vi "EXO2 Message.vi"(11 "字符串":string) -> (2 "数组":dbl[](array[numeric]), 3 "EXO message":T1)   [LabVIEW 2016, in "EXO2.lvlib"]
uses:
  EXO2.lvlib
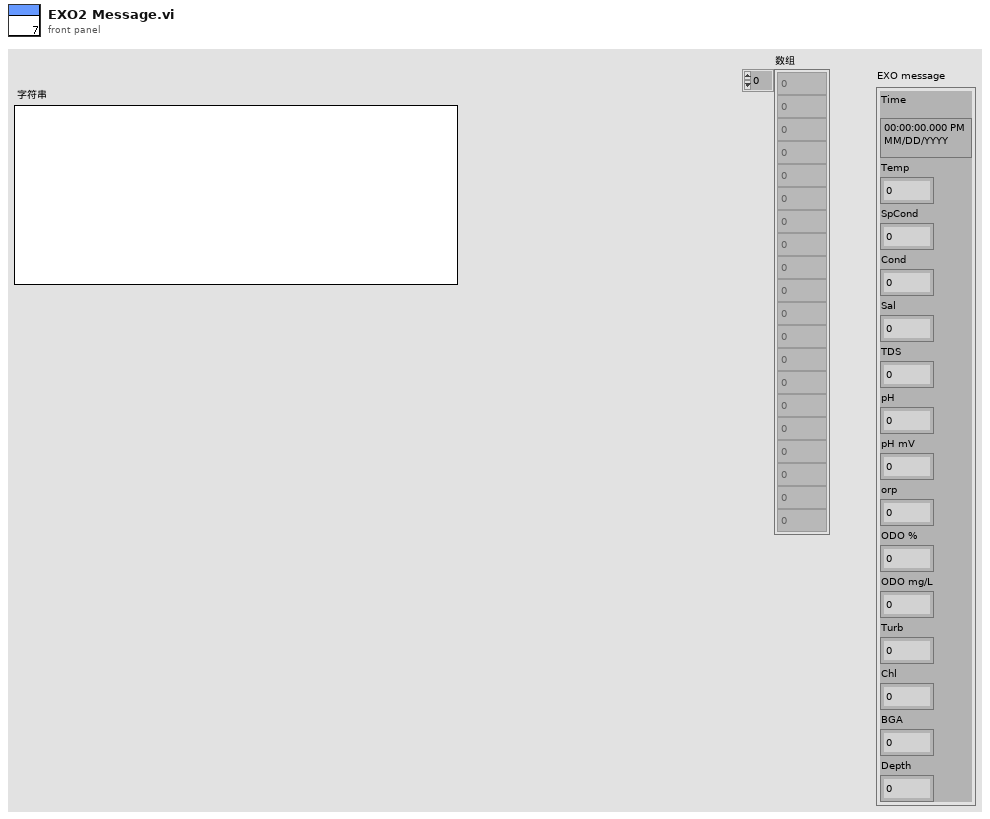
[diagram p1: front panel]
types:
  T1 = cluster{"Time":timestamp, "Temp":dbl, "SpCond":dbl, "Cond":dbl, "Sal":dbl, "TDS":dbl, "pH":dbl, "pH mV":dbl, "orp":dbl, "ODO %":dbl, "ODO mg/L":dbl, "Turb":dbl, "Chl":dbl, "BGA":dbl, "Depth":dbl}
  T2 = cluster{"seconds since 1Jan1904":timestamp, dbl, dbl, dbl, dbl, dbl, dbl, dbl, dbl, dbl, dbl, dbl, dbl, dbl, dbl}
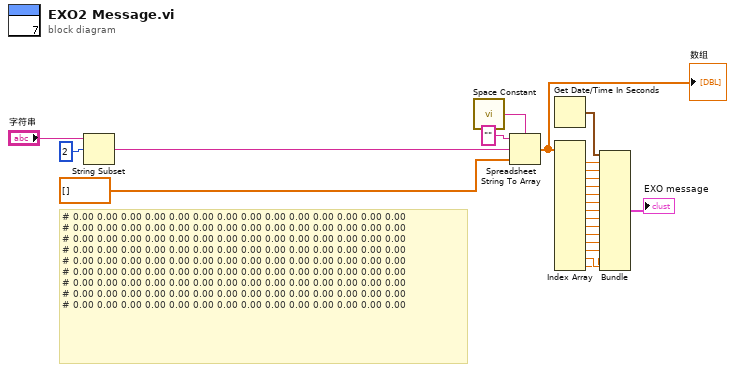
[diagram p0: block diagram]
diagram:
  # "# 0.00 0.00 0.00 0.00 0.00 0.00 0.00 0.00 0.00 0.00 0.00 0.00 0.00 0.00 \n# 0.00 0.00 0.00 0.00 0.00 0.00 0.00 0.00 0.00 0.00 0.00 0.00 0.00 0.00 \n# 0.00 0.00 0.00 0.00 0.00 0.00 0.00 0.00 0.00 0.00 0.00 0.00 0.00 0.00 \n# 0.00 0.00 0.00 0.00 0.00 0.00 0.00 0.00 0.00 0.00 0.00 0.00 0.00 0.00 \n# 0.00 0.00 0.00 0.00 0.00 0.00 0.00 0.00 0.00 0.00 0.00 0.00 0.00 0.00 \n# 0.00 0.00 0.00 0.00 0.00 0.00 0.00 0.00 0.00 0.00 0.00 0.00 0.00 0.00 \n# 0.00 0.00 0.00 0.00 0.00 0.00 0.00 0.00 0.00 0.00 0.00 0.00 0.00 0.00 \n# 0.00 0.00 0.00 0.00 0.00 0.00 0.00 0.00 0.00 0.00 0.00 0.00 0.00 0.00 \n# 0.00 0.00 0.00 0.00 0.00 0.00 0.00 0.00 0.00 0.00 0.00 0.00 0.00 0.00"
  n1 = String Subset(string="字符串", offset (0)=2 ("偏移量(0)")) -> (substring=w4:string)  [unwired: 1 in]
  n2 = call <vilib>:"Space Constant.vi"() -> ("String"=w23:string)
  n3 = Spreadsheet String To Array(delimiter (Tab)=w23, format string="" ("格式字符串"), spreadsheet string=w4, array type (2D Dbl)=dbl[] []) -> (array=w20:dbl[])
  "数组" <- w20
  n4 = Get Date/Time In Seconds() -> (seconds since 1Jan1904=w3:timestamp)
  n5 = Index Array(array=w20) -> (element #1=w19:dbl, element #2=w8:dbl, element #3=w9:dbl, element #4=w18:dbl, element #5=w17:dbl, element #6=w16:dbl, element #7=w15:dbl, element #8=w14:dbl, element #9=w13:dbl, element #10=w12:dbl, element #11=w11:dbl, element #12=w10:dbl, element #13=w2:dbl, element #14=w1:dbl)  [unwired: 14 in]
  n6 = Bundle("seconds since 1Jan1904"=w3, w19, w8, w9, w18, w17, w16, w15, w14, w13, w12, w11, w10, w1, w2) -> (→"EXO message":T2)  [unwired: 1 in]
